vi "Asylum_ReadString.vi"(8 "error in (no error)":errorcluster, 10 "parameterName":string, 11 "Application":refnum<k7>) -> (0 "error out":errorcluster, 3 "Application":refnum<k7>)   [LabVIEW 2016]
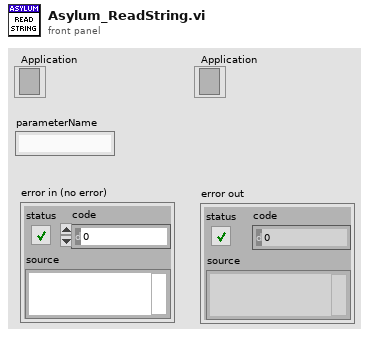
[diagram p1: front panel]
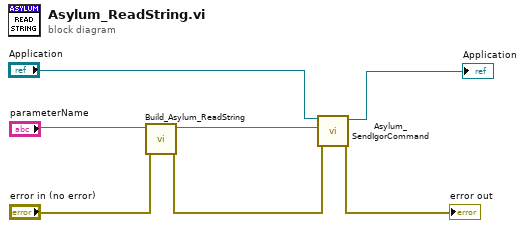
[diagram p0: block diagram]
diagram:
  n1 = call "Build_Asylum_ReadString.vi"("error in (no error)"="error in (no error)", "parameterName"="parameterName") -> ("error out"=w2:errorcluster, "String"=w6:string)  [unwired: 8 in]
  n2 = call "Asylum_SendIgorCommand.vi"("error in (no error)"=w2, "command"=w6, "Application"="Application") -> ("error out"=→"error out":errorcluster, "Application"=→"Application":refnum<k7>)  [unwired: 5 in, 2 out]
